vi "ShowErrorDBVI.vi"(8 "error in (no error)":errorcluster, 11 "DB in":refnum<class "DB.lvclass">) -> (0 "error out":errorcluster, 3 "DB out":refnum<class "DB.lvclass">)   [LabVIEW 2019, in "DB.lvclass"]
uses:
  DB.lvclass
  C:/Users/elysium/Documents/dev/TRANCON/Classes/GeneralFunctionality/GeneralFunctionality.lvclass
  GeneralFunctionality/GeneralFunctionality.lvclass/GeneralFunctionality.ctl
  GeneralFunctionality/GeneralFunctionality.lvclass
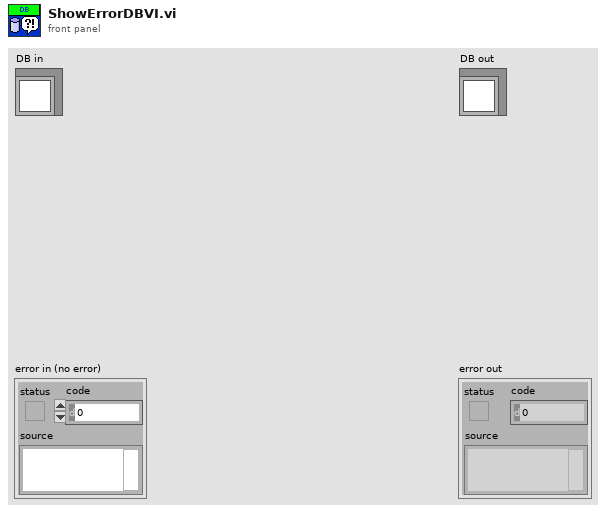
[diagram p1: front panel]
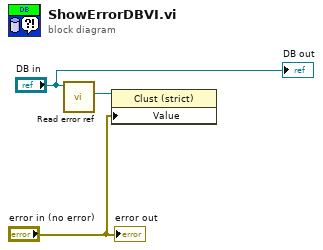
[diagram p0: block diagram]
diagram:
  n1 = call "Read error ref.vi"("GeneralFunctionality in"="DB in") -> ("error"=w2:refnum<vi>)  [unwired: 8 in, 2 out]
  n2 = property class="Clust (strict)"(reference=w2, "Value"="error in (no error)") -> ()  [unwired: 1 in, 2 out]
  "error out" <- "error in (no error)"
  "DB out" <- "DB in"
